vi "Start.vi"(8 "error in (no error)":errorcluster, 10 "Params":variant, 11 "PmuDelayClass in":refnum<class "FreqAnalysis.lvclass">) -> (0 "error out":errorcluster, 3 "PmuDelayClass out":refnum<class "FreqAnalysis.lvclass">)   [LabVIEW 2018, in "AnalysisPlugins.lvlib" / "FreqAnalysis.lvclass"]
uses:
  FreqAnalysis.lvclass
  C:/projects/ICDAS/NistPluggableModules/Analysis/AnalysisPlugins/AnalysisPluginBaseClass/AnalysisPluginsBase.lvclass
  C:/projects/ICDAS/NistPluggableModules/Analysis/AnalysisPlugins/FitterBaseClass/FitterBase.lvclass
  C:/projects/ICDAS/NistPluggableModules/Analysis/AnalysisPlugins/PmuAnalysisClass/PmuAnalysis.lvclass
  FGen/MemberClasses/PmuTestFunctions/Typedefs/PmuTestParams.ctl
  PmuAnalysisClass/PmuAnalysis.lvclass/PmuAnalysis.ctl
  FGen/MemberClasses/PmuTestFunctions/Typedefs/eParamIdx.ctl
  AnalysisPluginBaseClass/AnalysisPluginsBase.lvclass/AnalysisPluginsBase.ctl
  PmuAnalysisClass/Accessors/Read eTestType.vi
  AnalysisPluginBaseClass/Accessors/Write FileName.vi
  <vilib>/Utility/error.llb/Error Cluster From Error Code.vi
  <vilib>/ErrorRing/Error Ring.xnode
  FGen/MemberClasses/PmuTestFunctions/PmuTestFunctions.lvclass
  PmuAnalysisClass/PmuAnalysis.lvclass
  AnalysisPluginBaseClass/AnalysisPluginsBase.lvclass
  FitterBaseClass/FitterBase.lvclass
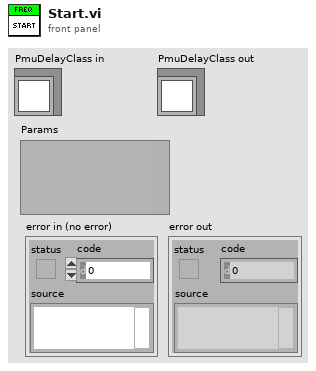
[diagram p1: front panel]
types:
  T1 = typedef "Functions.lvlib/PmuTestFunctions.lvclass/PmuTestParams.ctl" = dbl[][]
  T2 = typedef "Functions.lvlib/PmuTestFunctions.lvclass/eParamIdx.ctl" = enum16{"Xm", "Fin", "Ps", "Fh", "Ph", "Kh", "Fa", "Ka", "Fx", "Kx", "Rf", "KaS", "KxS", "KfS", "KrS"}
  T3 = enum16{"SteadyState", "Modulation", "Ramp", "Step"}
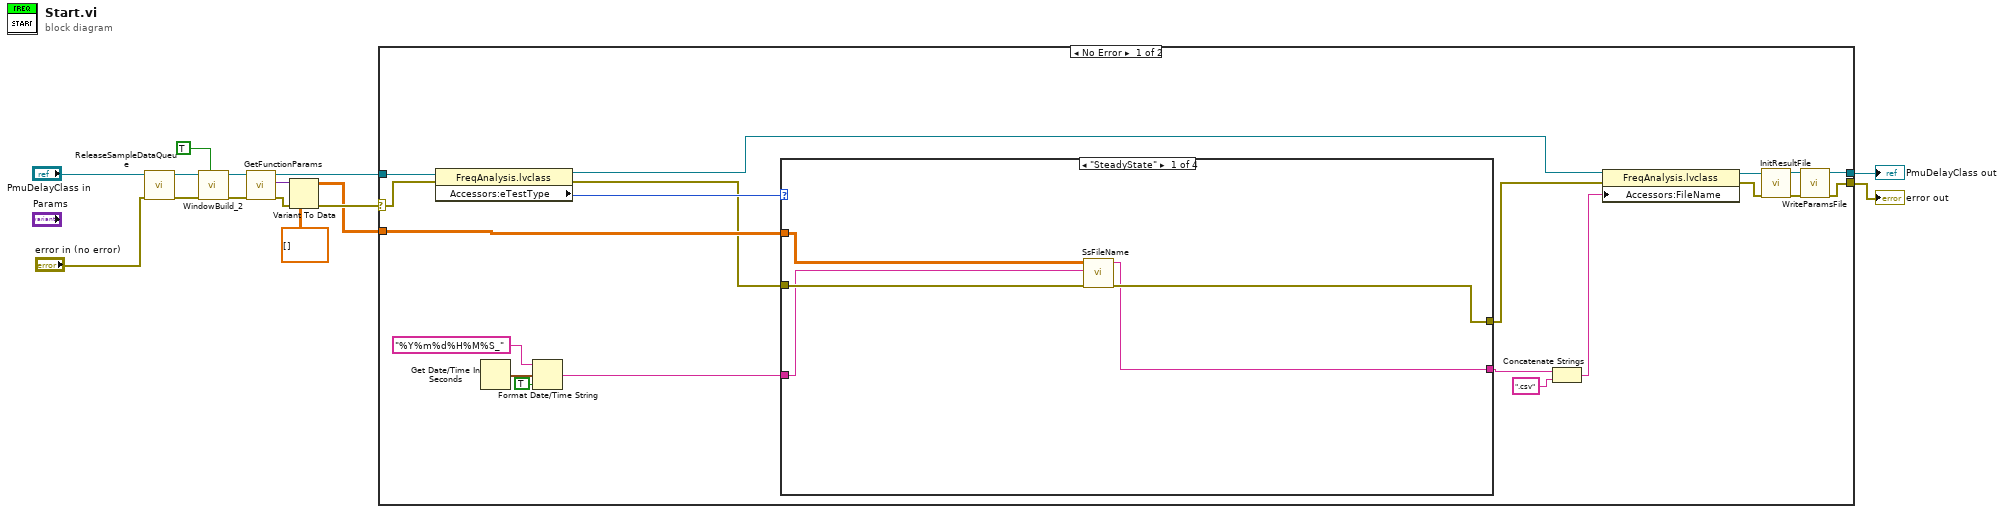
[diagram p0: block diagram]
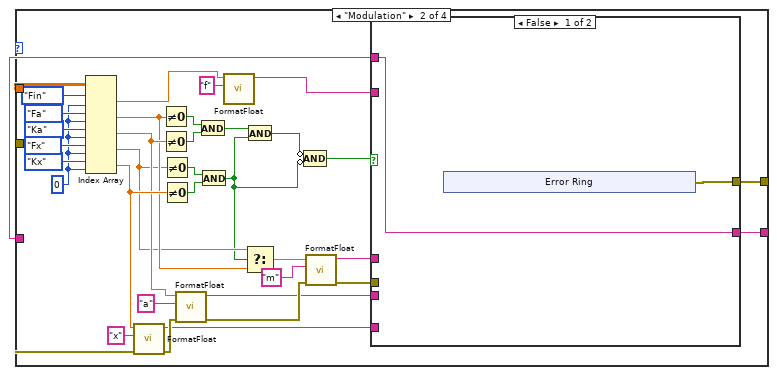
[diagram p2: hidden frame]
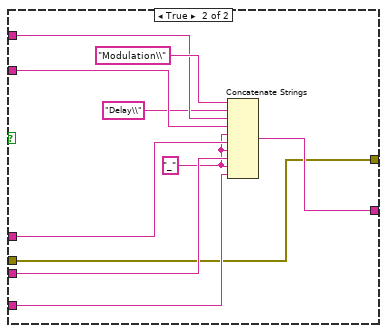
[diagram p3: hidden frame]
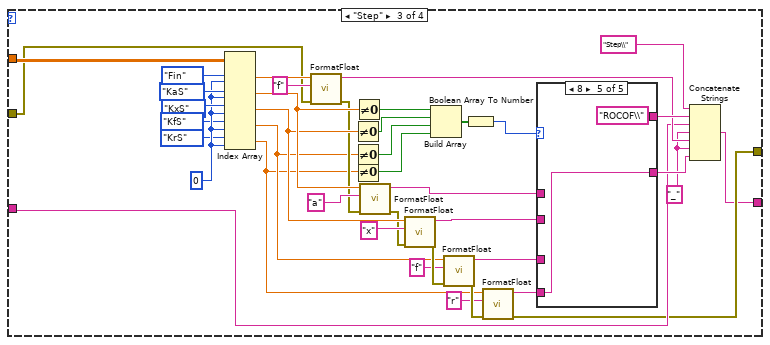
[diagram p4: hidden frame]
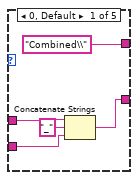
[diagram p5: hidden frame]
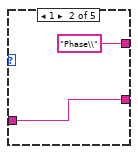
[diagram p6: hidden frame]
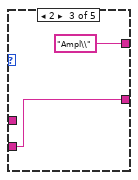
[diagram p7: hidden frame]
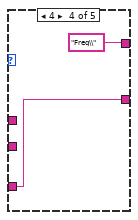
[diagram p8: hidden frame]
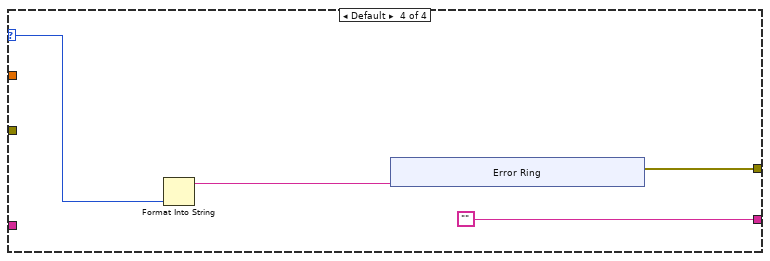
[diagram p9: hidden frame]
diagram:
  n1 = call "ReleaseSampleDataQueue.vi"("error in (no error)"="error in (no error)", "AnalysisPluginsBase in"="PmuDelayClass in") -> ("error out"=w6:errorcluster, "AnalysisPluginsBase out"=w5:refnum<class "FreqAnalysis.lvclass">)  [unwired: 8 in]
  n2 = call "WindowBuild_2.vi"("Init"=TRUE, "Error In"=w6, "Fitter in"=w5) -> ("Error Out"=w3:errorcluster, "Fitter out"=w4:refnum<class "FreqAnalysis.lvclass">)  [unwired: 6 in, 1 out]
  n3 = call-dynamic "GetFunctionParams.vi"("error in (no error)"=w3, "PmuAnalysis in"=w4) -> ("error out"=w14:errorcluster, "FunctionParams"=w15:variant, "PmuAnalysis out"=w11:refnum<class "FreqAnalysis.lvclass">)  [unwired: 7 in]
  n4 = Variant To Data(error in=w14, type=T1 [] ("Accessors:PmuTestParams"), Variant=w15) -> (data=w10:T1, error out=w12:errorcluster)
  n5 = case shown="No Error" w12 {
    selector: w12 -> [w34 w158]
    tunnel: w11 -> [w35 w159]
    tunnel: w10 -> [w29 _]
    tunnel: [w17 w159] -> w2
    tunnel: [w16 w158] -> w9
    frame No Error {
      n6 = property class="FreqAnalysis.lvclass"(reference=w35, error in=w34) -> (reference out=w26:refnum<class "FreqAnalysis.lvclass">, error out=w28:errorcluster, "Accessors:eTestType"=w30:T3)
      n7 = Get Date/Time In Seconds() -> (seconds since 1Jan1904=w32:timestamp)
      n8 = Format Date/Time String(time format string (%c)="%Y%m%d%H%M%S_", seconds (now)=w32, UTC format=TRUE) -> (date/time string=w27:string)
      n9 = case shown="\"SteadyState\"" w30 {
        selector: w30 -> [_ _ _ w149]
        tunnel: w28 -> [w40 w64 w97 _]
        tunnel: w29 -> [w39 w76 w98 _]
        tunnel: w27 -> [w38 w61 w96 _]
        tunnel: [w36 w55 w94 ""] -> w23
        tunnel: [w37 w41 w95 w148] -> w25
        frame "SteadyState" {
          n10 = call "SsFileName.vi"("error in (no error)"=w40, "Time"=w38, "Function Params"=w39) -> ("error out"=w37:errorcluster, "FileName"=w36:string)  [unwired: 7 in]
        }
        frame "Modulation" {
          w54 = 0 ("disabled index (col)")
          n11 = Index Array(array=w76, index (row) #1=eParamIdx."Fin" ("eParamIdx"), index (col) #1=w54, index (row) #2=eParamIdx."Fa" ("eParamIdx"), index (col) #2=w54, index (row) #3=eParamIdx."Ka" ("eParamIdx"), index (col) #3=w54, index (row) #4=eParamIdx."Fx" ("eParamIdx"), index (col) #4=w54, index (row) #5=eParamIdx."Kx" ("eParamIdx"), index (col) #5=w54) -> (element #1=w50:dbl, element #2=w47:dbl, element #3=w52:dbl, element #4=w46:dbl, element #5=w65:dbl)
          n12 = call "FormatFloat.vi"("error in (no error)"=w64, "replace string (\".\")"="x" ("replace string (\".\")"), "float"=w65) -> ("error out"=w62:errorcluster, "string"=w56:string)  [unwired: 7 in]
          n13 = Not Equal To 0?(x=w47) -> (x != 0?=w70:bool)
          n14 = Not Equal To 0?(x=w52) -> (x != 0?=w71:bool)
          n15 = Not Equal To 0?(x=w46) -> (x != 0?=w69:bool)
          n16 = Not Equal To 0?(x=w65) -> (x != 0?=w68:bool)
          n17 = call "FormatFloat.vi"("error in (no error)"=w62, "replace string (\".\")"="a" ("replace string (\".\")"), "float"=w52) -> ("error out"=w58:errorcluster, "string"=w57:string)  [unwired: 7 in]
          n18 = And(x=w70, y=w71) -> (x .and. y?=w67:bool)
          n19 = And(x=w69, y=w68) -> (x .and. y?=w44:bool)
          n20 = call "FormatFloat.vi"("replace string (\".\")"="f" ("replace string (\".\")"), "float"=w50) -> ("string"=w48:string)  [unwired: 8 in, 1 out]
          n21 = And(x=w67, y=w44) -> (x .and. y?=w45:bool)
          n22 = Select(t=w46, s=w44, f=w47) -> (s? t:f=w60:dbl)
          n23 = Compound Arithmetic op=AND(invert w45, invert w44) -> (w43:bool)
          n24 = call "FormatFloat.vi"("error in (no error)"=w58, "replace string (\".\")"="m" ("replace string (\".\")"), "float"=w60) -> ("error out"=w42:errorcluster, "string"=w49:string)  [unwired: 7 in]
          n25 = case shown="False" w43 {
            tunnel: w61 -> [w77 w92]
            tunnel: w57 -> [_ w91]
            tunnel: w56 -> [_ w90]
            tunnel: [w77 w89] -> w55
            tunnel: w49 -> [_ w88]
            tunnel: w48 -> [_ w87]
            tunnel: w42 -> [_ w84]
            tunnel: [w78 w84] -> w41
            frame False {
              n26 = xnode "Error Ring"() -> ("error out"=w78:errorcluster)
            }
            frame True {
              w86 = "_" ("string")
              n27 = Concatenate Strings("Modulation\\", "Delay\\", w92, w87, w86, w88, w86, w91, w86, w90) -> (w89:string)
            }
          }
        }
        frame "Step" {
          w112 = "_" ("string")
          w111 = 0 ("disabled index (col)")
          n28 = Index Array(array=w98, index (row) #1=eParamIdx."Fin" ("eParamIdx"), index (col) #1=w111, index (row) #2=eParamIdx."KaS" ("eParamIdx"), index (col) #2=w111, index (row) #3=eParamIdx."KxS" ("eParamIdx"), index (col) #3=w111, index (row) #4=eParamIdx."KfS" ("eParamIdx"), index (col) #4=w111, index (row) #5=eParamIdx."KrS" ("eParamIdx"), index (col) #5=w111) -> (element #1=w130:dbl, element #2=w128:dbl, element #3=w127:dbl, element #4=w104:dbl, element #5=w103:dbl)
          n29 = call "FormatFloat.vi"("error in (no error)"=w97, "replace string (\".\")"="f" ("replace string (\".\")"), "float"=w130) -> ("error out"=w124:errorcluster, "string"=w114:string)  [unwired: 7 in]
          n30 = Not Equal To 0?(x=w127) -> (x != 0?=w121:bool)
          n31 = Not Equal To 0?(x=w104) -> (x != 0?=w108:bool)
          n32 = Not Equal To 0?(x=w103) -> (x != 0?=w107:bool)
          n33 = Not Equal To 0?(x=w128) -> (x != 0?=w122:bool)
          n34 = call "FormatFloat.vi"("error in (no error)"=w124, "replace string (\".\")"="a" ("replace string (\".\")"), "float"=w128) -> ("error out"=w123:errorcluster, "string"=w118:string)  [unwired: 7 in]
          n35 = call "FormatFloat.vi"("error in (no error)"=w123, "replace string (\".\")"="x" ("replace string (\".\")"), "float"=w127) -> ("error out"=w106:errorcluster, "string"=w117:string)  [unwired: 7 in]
          n36 = Build Array(w122, w121, w108, w107) -> (w120:bool[])
          n37 = call "FormatFloat.vi"("error in (no error)"=w106, "replace string (\".\")"="f" ("replace string (\".\")"), "float"=w104) -> ("error out"=w105:errorcluster, "string"=w100:string)  [unwired: 7 in]
          n38 = Boolean Array To Number(Boolean array=w120) -> (number=w119:u32)
          n39 = call "FormatFloat.vi"("error in (no error)"=w105, "replace string (\".\")"="r" ("replace string (\".\")"), "float"=w103) -> ("error out"=w95:errorcluster, "string"=w99:string)  [unwired: 7 in]
          n40 = case shown="8" w119 {
            tunnel: ["Combined\\" "Phase\\" "Ampl\\" "Freq\\" "ROCOF\\"] -> w116
            tunnel: [w137 w139 w141 w143 w145] -> w113
            tunnel: w118 -> [w136 w139 _ _ _]
            tunnel: w117 -> [w134 _ w141 _ _]
            tunnel: w100 -> [_ _ _ w143 _]
            tunnel: w99 -> [_ _ _ _ w145]
            frame 0, Default {
              n41 = Concatenate Strings(w136, "_" ("string"), w134) -> (w137:string)
            }
            frame 1 {
            }
            frame 2 {
            }
            frame 4 {
            }
            frame 8 {
            }
          }
          n42 = Concatenate Strings("Step\\", w116, w96, w112, w114, w112, w113) -> (w94:string)
        }
        frame Default {
          n43 = Format Into String(w149) -> (resulting string=w150:string)  [unwired: 3 in, 1 out]
          n44 = xnode "Error Ring"("parameter 0"=w150) -> ("error out"=w148:errorcluster)
        }
      }
      n45 = Concatenate Strings(w23, ".csv" ("string")) -> (w22:string)
      n46 = property class="FreqAnalysis.lvclass"(reference=w26, error in=w25, "Accessors:FileName"=w22) -> (reference out=w21:refnum<class "FreqAnalysis.lvclass">, error out=w20:errorcluster)
      n47 = call-dynamic "InitResultFile.vi"("error in (no error)"=w20, "PmuDelayClass in"=w21) -> ("error out"=w18:errorcluster, "PmuDelayClass out"=w19:refnum<class "FreqAnalysis.lvclass">)  [unwired: 8 in]
      n48 = call "WriteParamsFile.vi"("error in (no error)"=w18, ":PmuAnalysis"=w19) -> ("error out"=w16:errorcluster, "PmuAnalysis"=w17:refnum<class "FreqAnalysis.lvclass">)  [unwired: 8 in]
    }
    frame Error {
    }
  }
  "error out" <- w9
  "PmuDelayClass out" <- w2
